vi "Recursive Get Size.vi"(11 "Control":refnum<vi>) -> (0 "error out":errorcluster, 3 "Size":T1)   [LabVIEW 2020, in "UIM.lvlib" / "SizeUIP.lvclass"]
uses:
  SizeUIP.lvclass
  <vilib>/Utility/miscctls.llb/LVBoundsTypeDef.ctl
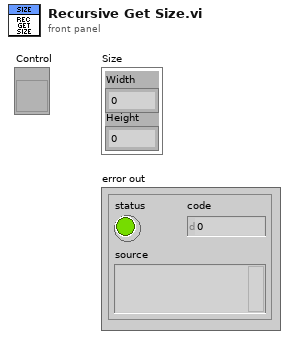
[diagram p1: front panel]
types:
  T1 = typedef "LVBoundsTypeDef.ctl" = cluster{"Width":u32, "Height":u32}
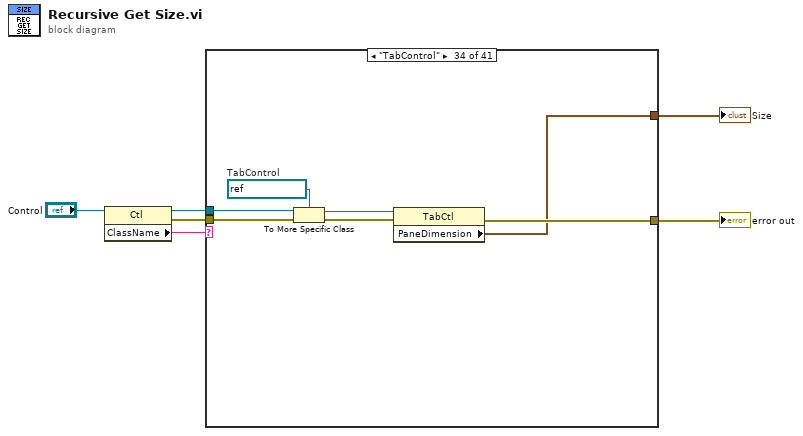
[diagram p0: block diagram]
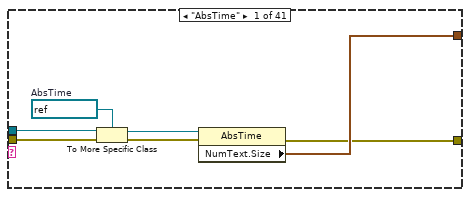
[diagram p2: hidden frame]
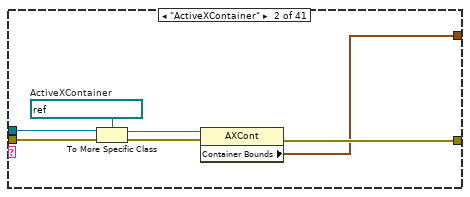
[diagram p3: hidden frame]
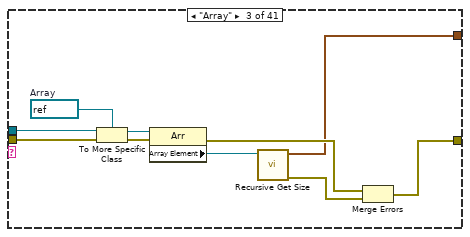
[diagram p4: hidden frame]
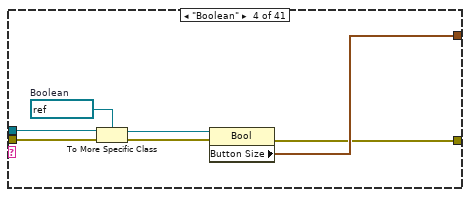
[diagram p5: hidden frame]
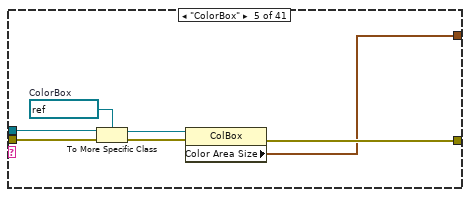
[diagram p6: hidden frame]
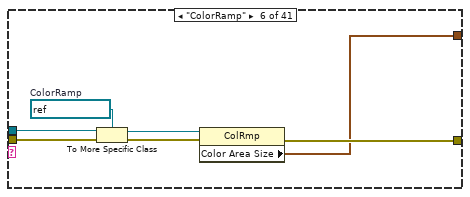
[diagram p7: hidden frame]
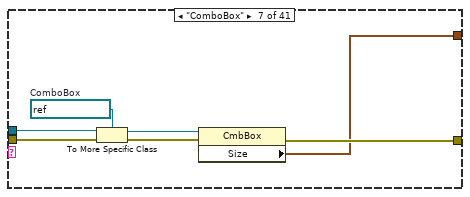
[diagram p8: hidden frame]
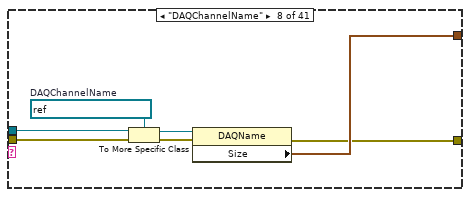
[diagram p9: hidden frame]
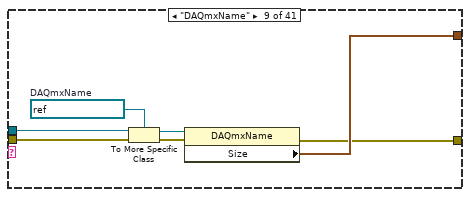
[diagram p10: hidden frame]
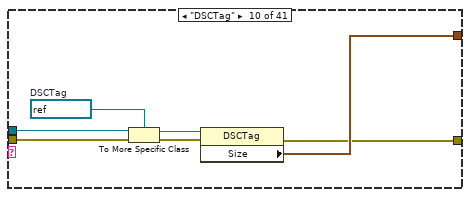
[diagram p11: hidden frame]
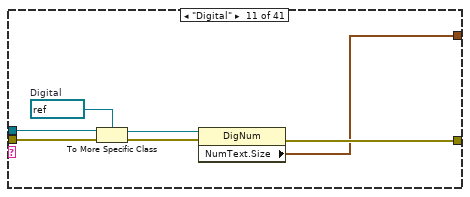
[diagram p12: hidden frame]
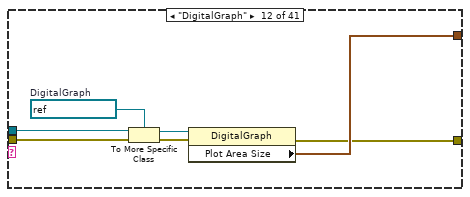
[diagram p13: hidden frame]
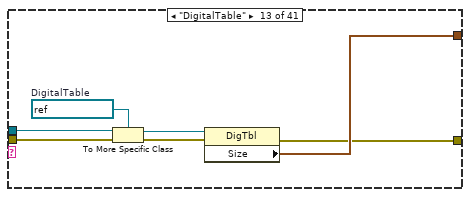
[diagram p14: hidden frame]
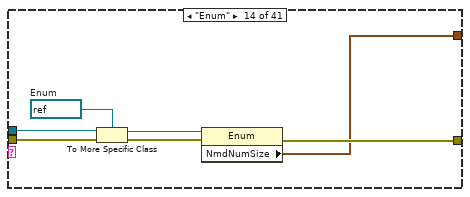
[diagram p15: hidden frame]
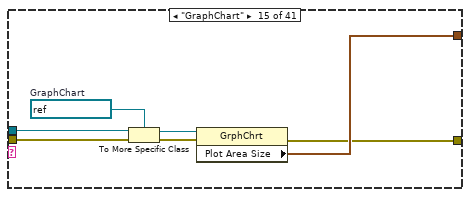
[diagram p16: hidden frame]
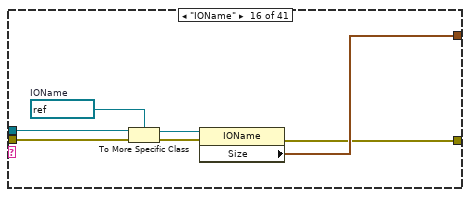
[diagram p17: hidden frame]
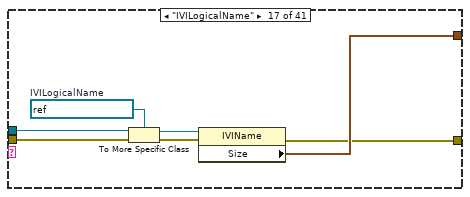
[diagram p18: hidden frame]
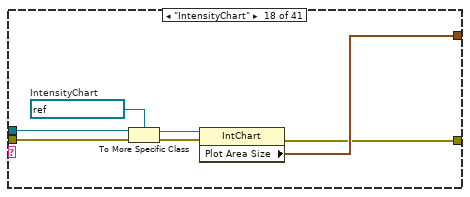
[diagram p19: hidden frame]
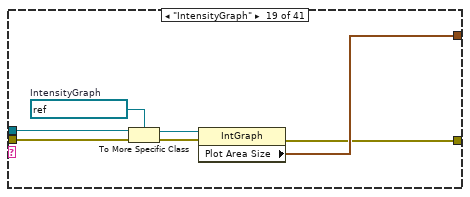
[diagram p20: hidden frame]
diagram:
  n1 = property class="Ctl"(reference="Control") -> (reference out=w4:refnum<vi>, error out=w3:errorcluster, "ClassName"=w2:string)  [unwired: 1 in]
  n2 = case shown="\"TabControl\"" w2 {
    tunnel: w3 -> [w13 w20 w30 w37 w44 w51 w58 w65 w72 w79 w86 w93 w100 w107 w114 w121 w128 w135 w142 w149 w156 w163 w170 w177 w184 w191 w198 w205 w212 w219 w226 w233 w240 w247 w254 w261 w268 w275 w282 w289 w290]
    tunnel: w4 -> [w12 w19 w29 w36 w43 w50 w57 w64 w71 w78 w85 w92 w99 w106 w113 w120 w127 w134 w141 w148 w155 w162 w169 w176 w183 w190 w197 w204 w211 w218 w225 w232 w239 w246 w253 w260 w267 w274 w281 w288 _]
    tunnel: [w8 w14 w21 w32 w38 w45 w52 w60 w67 w74 w80 w88 w95 w101 w109 w116 w123 w130 w137 w143 w150 w157 w165 w171 w178 w185 w192 w199 w206 w213 w220 w227 w234 w241 w248 w255 w263 w270 w277 w284 _] -> w5
    tunnel: [w7 w15 w22 w31 w39 w46 w53 w59 w66 w73 w81 w87 w94 w102 w108 w115 w122 w129 w136 w144 w151 w158 w164 w172 w179 w186 w193 w200 w207 w214 w221 w228 w235 w242 w249 w256 w262 w269 w276 w283 w290] -> w6
    frame "AbsTime" {
      w11 = refnum<vi> refnum  # AbsTime
      n3 = To More Specific Class(target class=w11, reference=w12, error in=w13) -> (specific class reference=w10:refnum<vi>, error out=w9:errorcluster)
      n4 = property class="AbsTime"(reference=w10, error in=w9) -> (error out=w7:errorcluster, "NumText.Size"=w8:T1)  [unwired: 1 out]
    }
    frame "ActiveXContainer" {
      w18 = refnum<vi> refnum  # ActiveXContainer
      n5 = To More Specific Class(target class=w18, reference=w19, error in=w20) -> (specific class reference=w17:refnum<vi>, error out=w16:errorcluster)
      n6 = property class="AXCont"(reference=w17, error in=w16) -> (error out=w15:errorcluster, "Container Bounds"=w14:T1)  [unwired: 1 out]
    }
    frame "Array" {
      w28 = refnum<vi> refnum  # Array
      n7 = To More Specific Class(target class=w28, reference=w29, error in=w30) -> (specific class reference=w27:refnum<vi>, error out=w26:errorcluster)
      n8 = property class="Arr"(reference=w27, error in=w26) -> (error out=w23:errorcluster, "Array Element"=w25:refnum<vi>)  [unwired: 1 out]
      n9 = call "Recursive Get Size.vi"("Control"=w25) -> ("error out"=w24:errorcluster, "Size"=w21:T1)  [unwired: 9 in]
      n10 = Merge Errors(w23, w24) -> (w22:errorcluster)
    }
    frame "Boolean" {
      w35 = refnum<vi> refnum  # Boolean
      n11 = To More Specific Class(target class=w35, reference=w36, error in=w37) -> (specific class reference=w34:refnum<vi>, error out=w33:errorcluster)
      n12 = property class="Bool"(reference=w34, error in=w33) -> (error out=w31:errorcluster, "Button Size"=w32:T1)  [unwired: 1 out]
    }
    frame "ColorBox" {
      w42 = refnum<vi> refnum  # ColorBox
      n13 = To More Specific Class(target class=w42, reference=w43, error in=w44) -> (specific class reference=w41:refnum<vi>, error out=w40:errorcluster)
      n14 = property class="ColBox"(reference=w41, error in=w40) -> (error out=w39:errorcluster, "Color Area Size"=w38:T1)  [unwired: 1 out]
    }
    frame "ColorRamp" {
      w49 = refnum<vi> refnum  # ColorRamp
      n15 = To More Specific Class(target class=w49, reference=w50, error in=w51) -> (specific class reference=w48:refnum<vi>, error out=w47:errorcluster)
      n16 = property class="ColRmp"(reference=w48, error in=w47) -> (error out=w46:errorcluster, "Color Area Size"=w45:T1)  [unwired: 1 out]
    }
    frame "ComboBox" {
      w56 = refnum<vi> refnum  # ComboBox
      n17 = To More Specific Class(target class=w56, reference=w57, error in=w58) -> (specific class reference=w55:refnum<vi>, error out=w54:errorcluster)
      n18 = property class="CmbBox"(reference=w55, error in=w54) -> (error out=w53:errorcluster, "Size"=w52:T1)  [unwired: 1 out]
    }
    frame "DAQChannelName" {
      w63 = refnum<vi> refnum  # DAQChannelName
      n19 = To More Specific Class(target class=w63, reference=w64, error in=w65) -> (specific class reference=w62:refnum<vi>, error out=w61:errorcluster)
      n20 = property class="DAQName"(reference=w62, error in=w61) -> (error out=w59:errorcluster, "Size"=w60:T1)  [unwired: 1 out]
    }
    frame "DAQmxName" {
      w70 = refnum<vi> refnum  # DAQmxName
      n21 = To More Specific Class(target class=w70, reference=w71, error in=w72) -> (specific class reference=w69:refnum<vi>, error out=w68:errorcluster)
      n22 = property class="DAQmxName"(reference=w69, error in=w68) -> (error out=w66:errorcluster, "Size"=w67:T1)  [unwired: 1 out]
    }
    frame "DSCTag" {
      w77 = refnum<vi> refnum  # DSCTag
      n23 = To More Specific Class(target class=w77, reference=w78, error in=w79) -> (specific class reference=w76:refnum<vi>, error out=w75:errorcluster)
      n24 = property class="DSCTag"(reference=w76, error in=w75) -> (error out=w73:errorcluster, "Size"=w74:T1)  [unwired: 1 out]
    }
    frame "Digital" {
      w84 = refnum<vi> refnum  # Digital
      n25 = To More Specific Class(target class=w84, reference=w85, error in=w86) -> (specific class reference=w83:refnum<vi>, error out=w82:errorcluster)
      n26 = property class="DigNum"(reference=w83, error in=w82) -> (error out=w81:errorcluster, "NumText.Size"=w80:T1)  [unwired: 1 out]
    }
    frame "DigitalGraph" {
      w91 = refnum<vi> refnum  # DigitalGraph
      n27 = To More Specific Class(target class=w91, reference=w92, error in=w93) -> (specific class reference=w90:refnum<vi>, error out=w89:errorcluster)
      n28 = property class="DigitalGraph"(reference=w90, error in=w89) -> (error out=w87:errorcluster, "Plot Area Size"=w88:T1)  [unwired: 1 out]
    }
    frame "DigitalTable" {
      w98 = refnum<vi> refnum  # DigitalTable
      n29 = To More Specific Class(target class=w98, reference=w99, error in=w100) -> (specific class reference=w97:refnum<vi>, error out=w96:errorcluster)
      n30 = property class="DigTbl"(reference=w97, error in=w96) -> (error out=w94:errorcluster, "Size"=w95:T1)  [unwired: 1 out]
    }
    frame "Enum" {
      w105 = refnum<vi> refnum  # Enum
      n31 = To More Specific Class(target class=w105, reference=w106, error in=w107) -> (specific class reference=w104:refnum<vi>, error out=w103:errorcluster)
      n32 = property class="Enum"(reference=w104, error in=w103) -> (error out=w102:errorcluster, "NmdNumSize"=w101:T1)  [unwired: 1 out]
    }
    frame "GraphChart" {
      w112 = refnum<vi> refnum  # GraphChart
      n33 = To More Specific Class(target class=w112, reference=w113, error in=w114) -> (specific class reference=w111:refnum<vi>, error out=w110:errorcluster)
      n34 = property class="GrphChrt"(reference=w111, error in=w110) -> (error out=w108:errorcluster, "Plot Area Size"=w109:T1)  [unwired: 1 out]
    }
    frame "IOName" {
      w119 = refnum<vi> refnum  # IOName
      n35 = To More Specific Class(target class=w119, reference=w120, error in=w121) -> (specific class reference=w118:refnum<vi>, error out=w117:errorcluster)
      n36 = property class="IOName"(reference=w118, error in=w117) -> (error out=w115:errorcluster, "Size"=w116:T1)  [unwired: 1 out]
    }
    frame "IVILogicalName" {
      w126 = refnum<vi> refnum  # IVILogicalName
      n37 = To More Specific Class(target class=w126, reference=w127, error in=w128) -> (specific class reference=w125:refnum<vi>, error out=w124:errorcluster)
      n38 = property class="IVIName"(reference=w125, error in=w124) -> (error out=w122:errorcluster, "Size"=w123:T1)  [unwired: 1 out]
    }
    frame "IntensityChart" {
      w133 = refnum<vi> refnum  # IntensityChart
      n39 = To More Specific Class(target class=w133, reference=w134, error in=w135) -> (specific class reference=w132:refnum<vi>, error out=w131:errorcluster)
      n40 = property class="IntChart"(reference=w132, error in=w131) -> (error out=w129:errorcluster, "Plot Area Size"=w130:T1)  [unwired: 1 out]
    }
    frame "IntensityGraph" {
      w140 = refnum<vi> refnum  # IntensityGraph
      n41 = To More Specific Class(target class=w140, reference=w141, error in=w142) -> (specific class reference=w139:refnum<vi>, error out=w138:errorcluster)
      n42 = property class="IntGraph"(reference=w139, error in=w138) -> (error out=w136:errorcluster, "Plot Area Size"=w137:T1)  [unwired: 1 out]
    }
    frame "Knob" {
      w147 = refnum<vi> refnum  # Knob
      n43 = To More Specific Class(target class=w147, reference=w148, error in=w149) -> (specific class reference=w146:refnum<vi>, error out=w145:errorcluster)
      n44 = property class="Knob"(reference=w146, error in=w145) -> (error out=w144:errorcluster, "Housing Size"=w143:T1)  [unwired: 1 out]
    }
    frame "ListBox" {
      w154 = refnum<vi> refnum  # ListBox
      n45 = To More Specific Class(target class=w154, reference=w155, error in=w156) -> (specific class reference=w153:refnum<vi>, error out=w152:errorcluster)
      n46 = property class="LstBox"(reference=w153, error in=w152) -> (error out=w151:errorcluster, "Size"=w150:T1)  [unwired: 1 out]
    }
    frame "MixedCheckbox" {
      w161 = refnum<vi> refnum  # MixedCheckbox
      n47 = To More Specific Class(target class=w161, reference=w162, error in=w163) -> (specific class reference=w160:refnum<vi>, error out=w159:errorcluster)
      n48 = property class="MixedCheckbox"(reference=w160, error in=w159) -> (error out=w158:errorcluster, "Text.Size"=w157:T1)  [unwired: 1 out]
    }
    frame "MixedSignalGraph" {
      w168 = refnum<vi> refnum  # MixedSignalGraph
      n49 = To More Specific Class(target class=w168, reference=w169, error in=w170) -> (specific class reference=w167:refnum<vi>, error out=w166:errorcluster)
      n50 = property class="MixedGraph"(reference=w167, error in=w166) -> (error out=w164:errorcluster, "Plot Area Size"=w165:T1)  [unwired: 1 out]
    }
    frame "MulticolumnListbox" {
      w175 = refnum<vi> refnum  # MulticolumnListbox
      n51 = To More Specific Class(target class=w175, reference=w176, error in=w177) -> (specific class reference=w174:refnum<vi>, error out=w173:errorcluster)
      n52 = property class="MCListbox"(reference=w174, error in=w173) -> (error out=w172:errorcluster, "Size"=w171:T1)  [unwired: 1 out]
    }
    frame "NamedNumeric" {
      w182 = refnum<vi> refnum  # NamedNumeric
      n53 = To More Specific Class(target class=w182, reference=w183, error in=w184) -> (specific class reference=w181:refnum<vi>, error out=w180:errorcluster)
      n54 = property class="NmdNum"(reference=w181, error in=w180) -> (error out=w179:errorcluster, "NmdNumSize"=w178:T1)  [unwired: 1 out]
    }
    frame "NumericWithScale" {
      w189 = refnum<vi> refnum  # NumericWithScale
      n55 = To More Specific Class(target class=w189, reference=w190, error in=w191) -> (specific class reference=w188:refnum<vi>, error out=w187:errorcluster)
      n56 = property class="NumWthScl"(reference=w188, error in=w187) -> (error out=w186:errorcluster, "Housing Size"=w185:T1)  [unwired: 1 out]
    }
    frame "Path" {
      w196 = refnum<vi> refnum  # Path
      n57 = To More Specific Class(target class=w196, reference=w197, error in=w198) -> (specific class reference=w195:refnum<vi>, error out=w194:errorcluster)
      n58 = property class="Path"(reference=w195, error in=w194) -> (error out=w193:errorcluster, "Size"=w192:T1)  [unwired: 1 out]
    }
    frame "Picture" {
      w203 = refnum<vi> refnum  # Picture
      n59 = To More Specific Class(target class=w203, reference=w204, error in=w205) -> (specific class reference=w202:refnum<vi>, error out=w201:errorcluster)
      n60 = property class="Pict"(reference=w202, error in=w201) -> (error out=w200:errorcluster, "Draw Area Size"=w199:T1)  [unwired: 1 out]
    }
    frame "Ring" {
      w210 = refnum<vi> refnum  # Ring
      n61 = To More Specific Class(target class=w210, reference=w211, error in=w212) -> (specific class reference=w209:refnum<vi>, error out=w208:errorcluster)
      n62 = property class="Ring"(reference=w209, error in=w208) -> (error out=w207:errorcluster, "NmdNumSize"=w206:T1)  [unwired: 1 out]
    }
    frame "SceneGraphDisplay" {
      w217 = refnum<vi> refnum  # SceneGraphDisplay
      n63 = To More Specific Class(target class=w217, reference=w218, error in=w219) -> (specific class reference=w216:refnum<vi>, error out=w215:errorcluster)
      n64 = property class="SceneGraphDisp"(reference=w216, error in=w215) -> (error out=w214:errorcluster, "ContentBounds"=w213:T1)  [unwired: 1 out]
    }
    frame "Slide" {
      w224 = refnum<vi> refnum  # Slide
      n65 = To More Specific Class(target class=w224, reference=w225, error in=w226) -> (specific class reference=w223:refnum<vi>, error out=w222:errorcluster)
      n66 = property class="Slide"(reference=w223, error in=w222) -> (error out=w221:errorcluster, "Housing Size"=w220:T1)  [unwired: 1 out]
    }
    frame "String" {
      w231 = refnum<vi> refnum  # String
      n67 = To More Specific Class(target class=w231, reference=w232, error in=w233) -> (specific class reference=w230:refnum<vi>, error out=w229:errorcluster)
      n68 = property class="Str"(reference=w230, error in=w229) -> (error out=w228:errorcluster, "Size"=w227:T1)  [unwired: 1 out]
    }
    frame "SubPanel" {
      w238 = refnum<vi> refnum  # SubPanel
      n69 = To More Specific Class(target class=w238, reference=w239, error in=w240) -> (specific class reference=w237:refnum<vi>, error out=w236:errorcluster)
      n70 = property class="SubPnl"(reference=w237, error in=w236) -> (error out=w235:errorcluster, "Container Bounds"=w234:T1)  [unwired: 1 out]
    }
    frame "TabControl" {
      w245 = refnum<vi> refnum  # TabControl
      n71 = To More Specific Class(target class=w245, reference=w246, error in=w247) -> (specific class reference=w244:refnum<vi>, error out=w243:errorcluster)
      n72 = property class="TabCtl"(reference=w244, error in=w243) -> (error out=w242:errorcluster, "PaneDimension"=w241:T1)  [unwired: 1 out]
    }
    frame "Table" {
      w252 = refnum<vi> refnum  # Table
      n73 = To More Specific Class(target class=w252, reference=w253, error in=w254) -> (specific class reference=w251:refnum<vi>, error out=w250:errorcluster)
      n74 = property class="Tbl"(reference=w251, error in=w250) -> (error out=w249:errorcluster, "Size"=w248:T1)  [unwired: 1 out]
    }
    frame "TreeControl" {
      w259 = refnum<vi> refnum  # TreeControl
      n75 = To More Specific Class(target class=w259, reference=w260, error in=w261) -> (specific class reference=w258:refnum<vi>, error out=w257:errorcluster)
      n76 = property class="Tree"(reference=w258, error in=w257) -> (error out=w256:errorcluster, "Size"=w255:T1)  [unwired: 1 out]
    }
    frame "VISAResourceName" {
      w266 = refnum<vi> refnum  # VISAResourceName
      n77 = To More Specific Class(target class=w266, reference=w267, error in=w268) -> (specific class reference=w265:refnum<vi>, error out=w264:errorcluster)
      n78 = property class="VISAName"(reference=w265, error in=w264) -> (error out=w262:errorcluster, "Size"=w263:T1)  [unwired: 1 out]
    }
    frame "WaveformChart" {
      w273 = refnum<vi> refnum  # WaveformChart
      n79 = To More Specific Class(target class=w273, reference=w274, error in=w275) -> (specific class reference=w272:refnum<vi>, error out=w271:errorcluster)
      n80 = property class="WFChart"(reference=w272, error in=w271) -> (error out=w269:errorcluster, "Plot Area Size"=w270:T1)  [unwired: 1 out]
    }
    frame "WaveformGraph" {
      w280 = refnum<vi> refnum  # WaveformGraph
      n81 = To More Specific Class(target class=w280, reference=w281, error in=w282) -> (specific class reference=w279:refnum<vi>, error out=w278:errorcluster)
      n82 = property class="WFGraph"(reference=w279, error in=w278) -> (error out=w276:errorcluster, "Plot Area Size"=w277:T1)  [unwired: 1 out]
    }
    frame "XYGraph" {
      w287 = refnum<vi> refnum  # XYGraph
      n83 = To More Specific Class(target class=w287, reference=w288, error in=w289) -> (specific class reference=w286:refnum<vi>, error out=w285:errorcluster)
      n84 = property class="XYGraph"(reference=w286, error in=w285) -> (error out=w283:errorcluster, "Plot Area Size"=w284:T1)  [unwired: 1 out]
    }
    frame Default {
    }
  }
  "error out" <- w6
  "Size" <- w5
